vi "ma_Linear Averaging Done.vi"(1 "averaging parameters":T1={"averaging mode"=enum."No averaging", "weighting mode"=enum."Linear", "number of averages"=10} {"number of averages" min=1}, 2 "averaging done":bool) -> (0 "linear averaging done":bool)   [LabVIEW 2020, in "NI_MAPro.lvlib"]
uses:
  NI_MAPro.lvlib
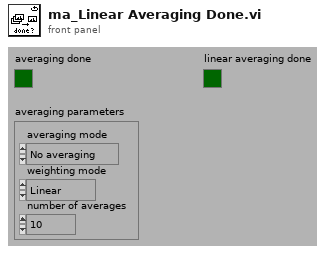
[diagram p1: front panel]
types:
  T1 = cluster{"averaging mode":enum16{"No averaging", "Vector averaging", "RMS averaging", "Peak hold"}, "weighting mode":enum16{"Linear", "Exponential"}, "number of averages":u32}
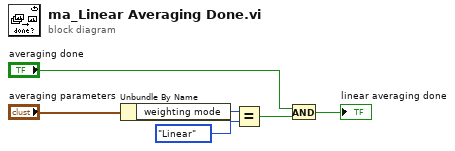
[diagram p0: block diagram]
diagram:
  n1 = Unbundle By Name("averaging parameters") -> ("weighting mode"=w4:enum16{"Linear", "Exponential"})
  n2 = Equal?(x=w4, y=enum16{"Linear", "Exponential"}."Linear") -> (x = y?=w6:bool)
  n3 = And(x="averaging done", y=w6) -> (x .and. y?=→"linear averaging done":bool)
